vi "DIOGet+.vi"(8 "error in (no error)":errorcluster, 10 "Sensor Type":enum16{"Active Low", "Active High"}(ring)=enum."Active High", 11 "DigitalInputDevRefIn":T1) -> (0 "error out":errorcluster, 2 "Value":bool, 3 "DigitalInputDevRefOut":T1)   [LabVIEW 2013]
uses:
  <vilib>/Rock Robotics/WPI/DigitalInput/WPI_DigitalInputDevRef.ctl
  <vilib>/Rock Robotics/SystemInterfaces/DIO/FPGA_DIOChannel.ctl
  <vilib>/Rock Robotics/SystemInterfaces/Typedef/FPGA_TypedefDigitalModule.ctl
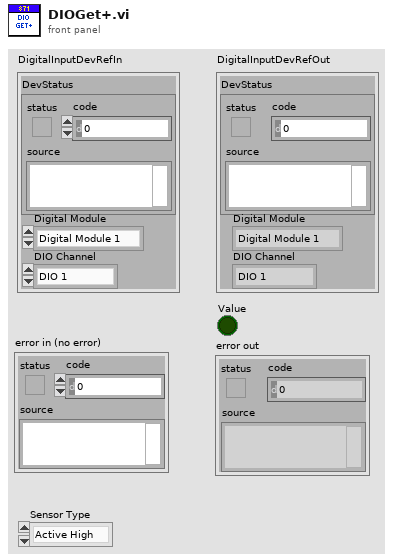
[diagram p1: front panel]
types:
  T1 = typedef "WPI_DigitalInputDevRef.ctl" = cluster{"DevStatus":errorcluster, "DIO Channel":T2, "Digital Module":T3}
  T2 = typedef "FPGA_DIOChannel.ctl" = enum8{"DIO 1", "DIO 2", "DIO 3", "DIO 4", "DIO 5", "DIO 6", "DIO 7", "DIO 8", "DIO 9", "DIO 10", "DIO 11", "DIO 12", "DIO 13", "DIO 14", "Invalid"}
  T3 = typedef "FPGA_TypedefDigitalModule.ctl" = enum16{"Digital Module 1", "Digital Module 2"}
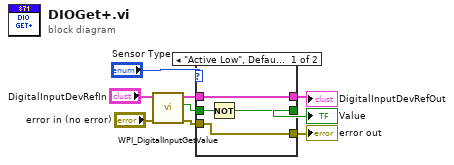
[diagram p0: block diagram]
diagram:
  n1 = call <vilib>:"WPI_DigitalInputGetValue.vi"("error in (no error)"="error in (no error)", "DigitalInputDevRef"="DigitalInputDevRefIn") -> ("error out"=w1:errorcluster, "Value"=w4:bool, "DigitalInputDevRef"=w5:T1)  [unwired: 7 in]
  n2 = case shown="\"Active Low\", Default" "Sensor Type" {
    tunnel: [w13 w16] -> w6
    tunnel: w5 -> [w13 w16]
    tunnel: w4 -> [w12 w15]
    tunnel: [w11 w15] -> w3
    tunnel: [w10 w14] -> w2
    tunnel: w1 -> [w10 w14]
    frame "Active Low", Default {
      n3 = Not(x=w12) -> (.not. x?=w11:bool)
    }
    frame "Active High" {
    }
  }
  "DigitalInputDevRefOut" <- w6
  "error out" <- w2
  "Value" <- w3
